vi "Pfeiffer Vacuum Turbo Config A D input output.vi"(8 "error in (no error)":errorcluster, 9 "PV config A D input output - Cluster":T1={"Parameter"=enum." Configuration DO2 (019)", "Parameter\nread only<->describe"=FALSE, "off<->on   "=TRUE, "Configuration DO1 / DO2 / R1 / R2 / R3"=0, "Configuration AO1"=0, "Config. Acces. A1/A2"=0, "Config. Acces. B1/B2"=0, "Configuration DI1 / DI2 / DI3"=0} {"Configuration DI1 / DI2 / DI3" items=["0 = deactivated", "1 = enable venting", "2 = heating", "3 = sealing gas", "4 = run-up time control", "5 = rotation speed setting mode", "6 =", "7 = Sensor 1 HV enable"]; "Config. Acces. B1/B2" items=[" fan (continous operation) (default)", " venting valve, normally closed", " heating", " backing pump", " fan (temperature controlled)", " sealing gas", " always 0 (off)", " always 1 (on)", " power failure venting unit"]; "Config. Acces. A1/A2" items=[" fan (continous operation)", " venting valve, normally closed", " heating", " backing pump", " fan (temperature controlled)", " sealing gas", " always off", " always on", " power failure venting unit"]; "Configuration DO1 / DO2 / R1 / R2 / R3" items=["0 = rot. speed switch point attained", "1 = no error", "2 = error", "3 = warning", "4 = error and/or warning", "5 = set speed attained", "6 = pump on", "7 = pump accelerates", "8 = pump decelerater", "9 = always 0 (off)", "10 = always 1 (on)", "11 = remote priority active", "12 = heating", "13 = backing pump", "14 = sealing gas", "15 = pumping station", "16 = pump rotates", "17 = pump does not rotate", "18 = TMS temperature engaged  ", "19 = Pressure below pressure switchpoint 1", "20 = Pressure below pressure switchpoint 2"]; "Configuration AO1" items=["0 = actual rotation speed", "1 = power", "2 = current", "3 = always 0 V", "4 = always 10 V", "5 = follows AI1", "6 = Pressure value 1", "7 = Pressure value 2"]}, 10 "Adress of unit":u16=1 min=1 max=999 step=1, 11 "COM Port Name in":refnum<visa-resource-name>="COM1") -> (0 "error out":errorcluster, 3 "response (data)":string)   [LabVIEW 2021]
doc: "There are 15 parameters available, only one of which can be enabled at a time. \n\n Configuration DO2 (019)\n Configuration DO1 (024) \n Configuration heating output (032)\n Configuration accessory A1 (035)\n Configuration accessory B1 (036)\n Configuration accessory A2 (037)\n Configuration accessory B2 (038)\n Configuration Relais 1 (045)\n Configuration Relais 2 (046)\n Configuration Relais 3 (047)\n Configuration AO1 (055)\n Configuration AI1 (057)\n Configuration DI1 (062)\n Configuration DI2 (063)\n Configuration DI3 (064)\n\nNote: The controls right of this one will set the appropriate values for the selected parameter. Any settings for an parameter that is not selected will be ignored. If a value is out of range, it will be changed to either the upper or the lower limit of the range."
uses:
  <instrlib>/Pfeiffer Vacuum/Public/Turbopumps/PV config A D input output - Cluster.ctl
  <instrlib>/Pfeiffer Vacuum/Pfeiffer Vacuum.lvlib
panel:
  # "<--------------                  ------------->     \n                                                                                        false                             true \n Configuration heating output K4    :                           heat/TMS            ealing gas valve control  \n Configuration AI 1                          :                            disabled                       set speed"
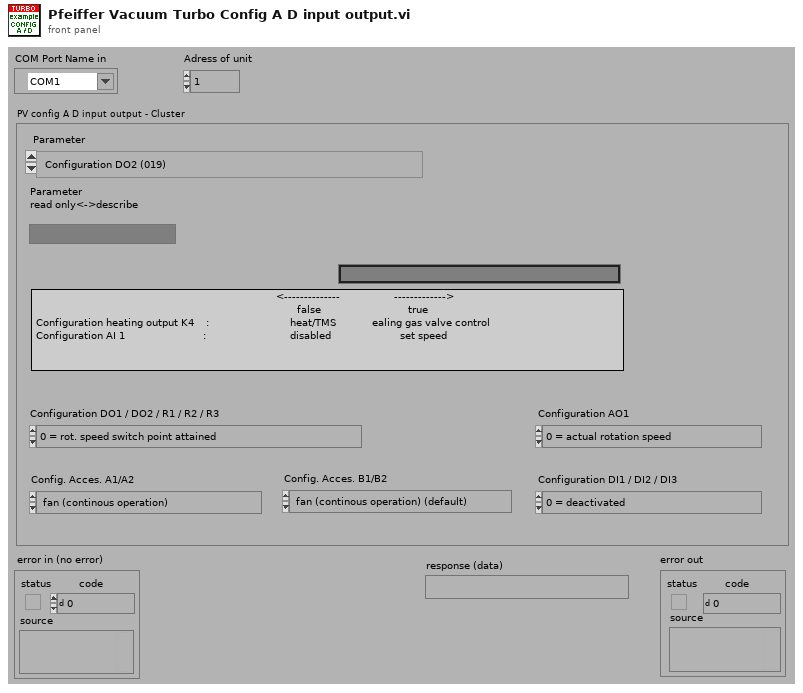
[diagram p1: front panel]
types:
  T1 = typedef "Pfeiffer Vacuum.lvlib/PV config A D input output - Cluster.ctl" = cluster{"Parameter":enum16{" Configuration DO2 (019)", " Configuration DO1 (024)", " Configuration heating output (032)", " Configuration accessory A1 (035)", " Configuration accessory B1 (036)", " Configuration accessory A2 (037)", " Configuration accessory B2 (038)", " Configuration Relais 1 (045)", " Configuration Relais 2 (046)", " Configuration Relais 3 (047)", " Configuration AO1 (055)", " Configuration AI1 (057)", " Configuration DI1 (062)", " Configuration DI2 (063)", " Configuration DI3 (064)"}, "Parameter\nread only<->describe":bool, "off<->on   ":bool, "Configuration DO1 / DO2 / R1 / R2 / R3":u16, "Configuration AO1":u16, "Config. Acces. A1/A2":u16, "Config. Acces. B1/B2":u16, "Configuration DI1 / DI2 / DI3":u16}
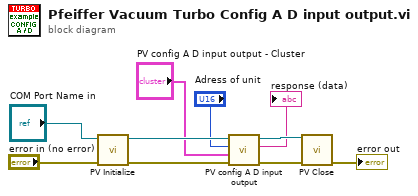
[diagram p0: block diagram]
diagram:
  n1 = call <instrlib>:"PV Initialize.vi"("error in (no error)"="error in (no error)", "VISA session in"="COM Port Name in") -> ("error out"=w10:errorcluster, "VISA session out"=w8:refnum<visa-resource-name>)  [unwired: 8 in]
  n2 = call <instrlib>:"PV config A D input output.vi"("error in (no error)"=w10, "PV config A D input output - Cluster"="PV config A D input output - Cluster", "Adress of unit"="Adress of unit", "VISA session"=w8) -> ("error out"=w9:errorcluster, "response (data)"=→"response (data)":string, "dup VISA session"=w7:refnum<visa-resource-name>)  [unwired: 5 in]
  n3 = call <instrlib>:"PV Close.vi"("VISA session"=w7, "error in (no error)"=w9) -> ("error out"=→"error out":errorcluster)  [unwired: 13 in]
